vi "Add_Orig_results_filename.vi"() -> ()   [LabVIEW 2010]
uses:
  Controls/File_Selector_Type.ctl
panel:
  in  "Previous Choice":path
  out "Files Processed":i32(slide) scale=0.0..95.0
  out "Current Filename":path
  in  "Search String":string
  in  "At Dialog Prompt Add Metadata to:":T1
  in  "stop":bool
  out "Index":i32=22
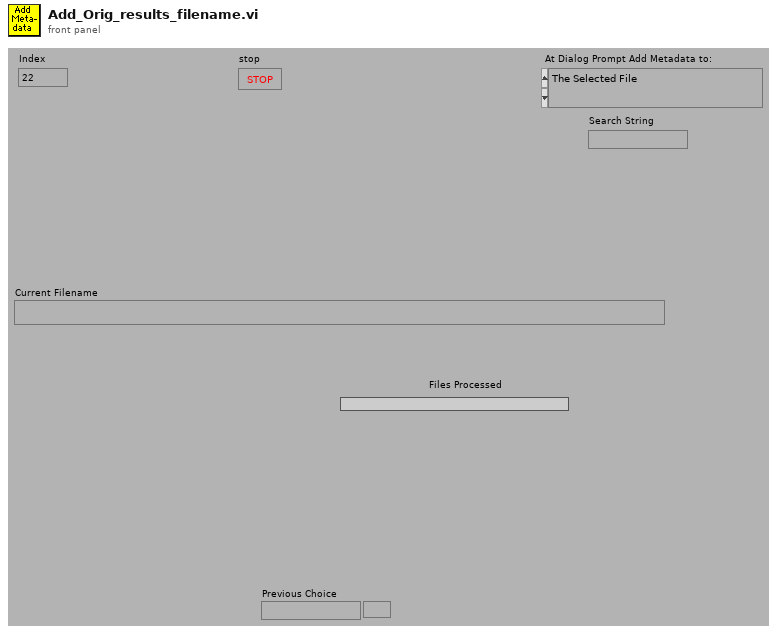
[diagram p1: front panel]
types:
  T1 = typedef "File_Selector_Type.ctl" = enum16{"The Selected File", "The Selected Folder", "Files containing the search string in the selected folder", "All files listed in selected file"}
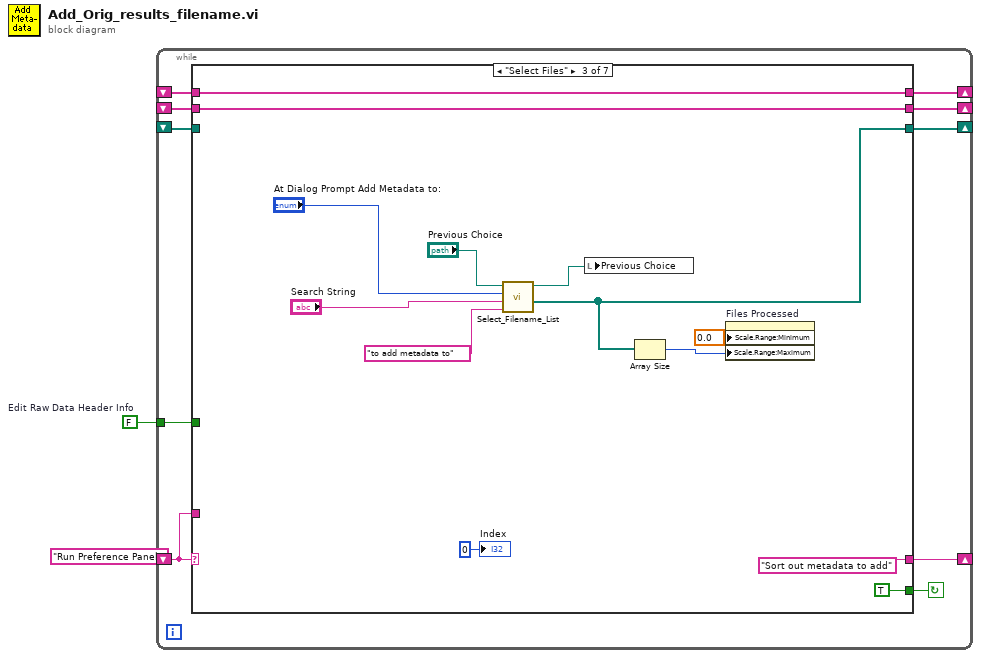
[diagram p0: block diagram]
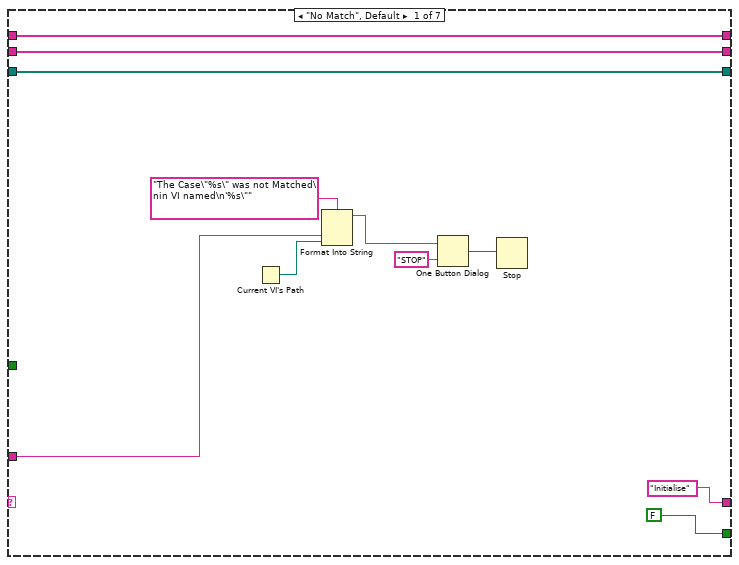
[diagram p2: hidden frame]
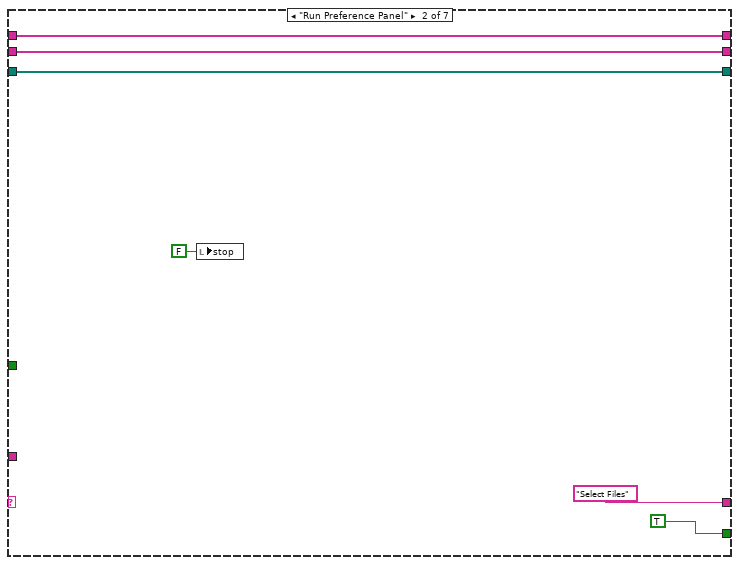
[diagram p3: hidden frame]
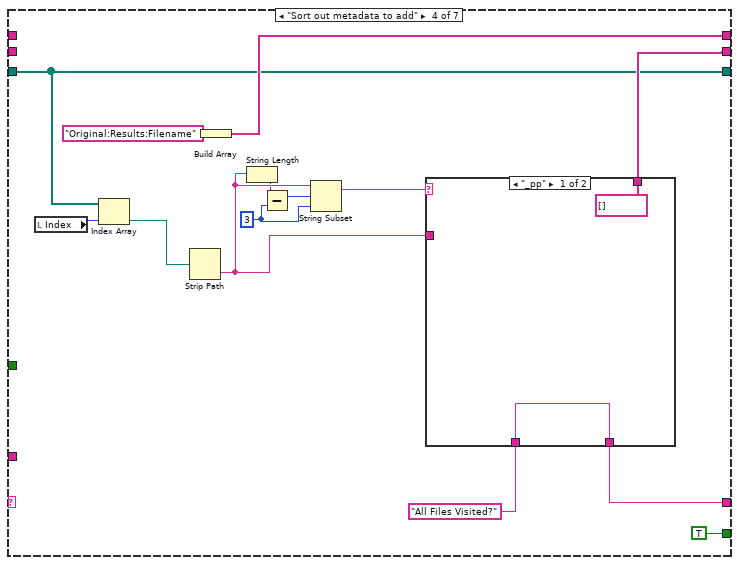
[diagram p4: hidden frame]
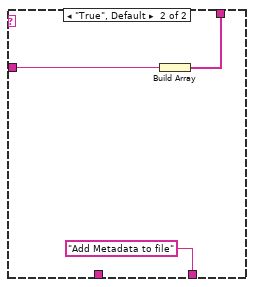
[diagram p5: hidden frame]
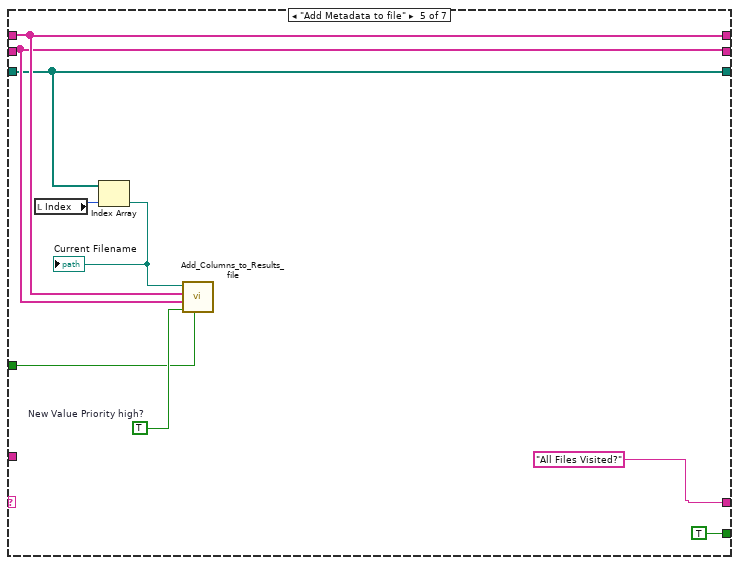
[diagram p6: hidden frame]
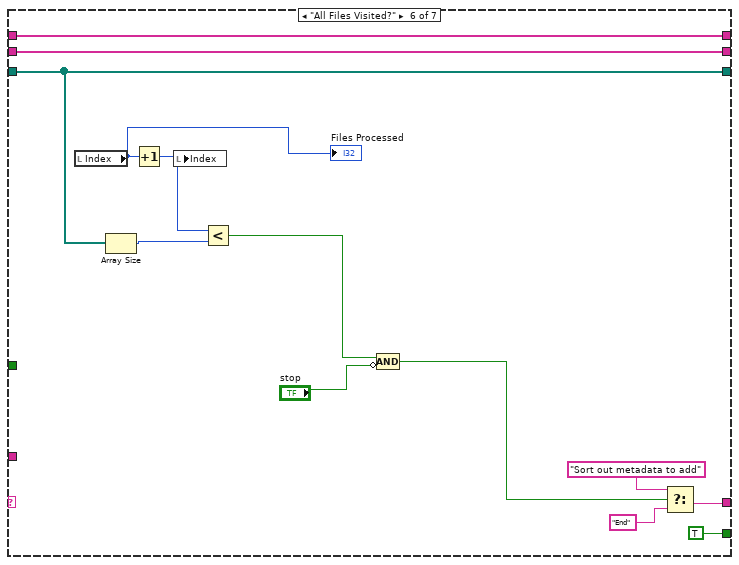
[diagram p7: hidden frame]
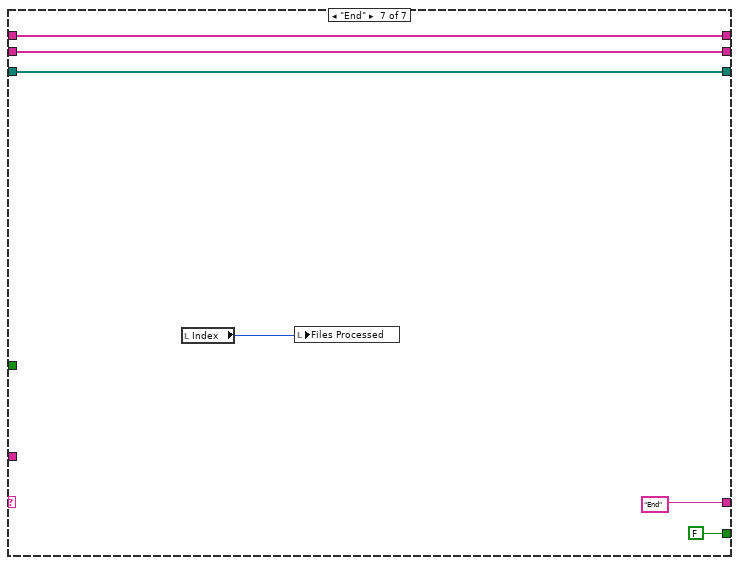
[diagram p8: hidden frame]
diagram:
  w1 = FALSE  # Edit Raw Data Header Info
  n1 = while {
    tunnel: w1 -> [w3]
    shift-left: _ -> [w4]
    shift-right: [w5] -> _
    shift-left: _ -> [w7]
    shift-right: [w6] -> _
    shift-left: _ -> [w9]
    shift-right: [w10] -> _
    shift-left: "Run Preference Panel" -> [w11]
    shift-right: [w12] -> _
    stop <- w8 continue-if-true
    n2 = case shown="\"Select Files\"" w11 {
      tunnel: [FALSE TRUE TRUE TRUE TRUE TRUE FALSE] -> w8
      tunnel: ["Initialise" "Select Files" "Sort out metadata to add" w52 "All Files Visited?" w71 "End"] -> w12
      tunnel: w11 -> [w18 _ _ _ _ _ _]
      tunnel: [w15 w28 w34 w50 w63 w83 w86] -> w10
      tunnel: w9 -> [w15 w28 _ w50 w63 w83 w86]
      tunnel: w7 -> [w14 w26 w37 _ w66 w78 w89]
      tunnel: [w14 w26 w37 w54 w66 w78 w89] -> w6
      tunnel: [w13 w25 w41 w53 w65 w77 w88] -> w5
      tunnel: w4 -> [w13 w25 w41 _ w65 w77 w88]
      tunnel: w3 -> [_ _ _ _ w64 _ _]
      frame "No Match", Default {
        n3 = Current VI's Path() -> (path=w17:path)
        n4 = Format Into String(format string="The Case\"%s\" was not Matched\nin VI named\n'%s\"" ("Format String"), w18, w17) -> (resulting string=w21:string)  [unwired: 2 in, 1 out]
        n5 = One Button Dialog(message=w21, button name ("OK")="STOP") -> (true=w19:bool)
        n6 = Stop(stop? (T)=w19) -> ()
      }
      frame "Run Preference Panel" {
        n7 = local write "stop"(FALSE ("stop")) -> ()
      }
      frame "Select Files" {
        n8 = call "Select_Filename_List.vi"("File Type"="to add metadata to", "Search String"="Search String", "At Dialog Prompt Post Process"="At Dialog Prompt Add Metadata to:", "Previous Choice"="Previous Choice") -> ("Selected files"=w34:path[], "Choosen path"=w31:path)  [unwired: 2 in, 1 out]
        n9 = local write "Previous Choice"(w31) -> ()
        n10 = Array Size(array=w34) -> (size(s)=w33:i32)
        n11 = property on="Files Processed" class="Slide (strict)"("Scale.Range:Minimum"=0.0, "Scale.Range:Maximum"=w33) -> ()  [unwired: 2 in, 2 out]
        "Index" <- 0 ("Index")
      }
      frame "Sort out metadata to add" {
        w45 = 3 ("length (rest)")
        n12 = local read "Index"() -> (w55:i32)
        n13 = Index Array(array=w50, index=w55) -> (element=w49:path)
        n14 = Strip Path(path=w49) -> (name=w47:string)  [unwired: 1 out]
        n15 = Build Array("Original:Results:Filename") -> (w54:string[])
        n16 = String Length(string=w47) -> (length=w46:i32)
        n17 = Subtract(x=w46, y=w45) -> (x-y=w44:i32)
        n18 = String Subset(string=w47, offset (0)=w44, length (rest)=w45) -> (substring=w43:string)
        n19 = case shown="\"_pp\"" w43 {
          tunnel: [string[] [] w59] -> w53
          tunnel: [w57 "Add Metadata to file"] -> w52
          tunnel: "All Files Visited?" -> [w57 _]
          tunnel: w47 -> [_ w60]
          frame "_pp" {
          }
          frame "True", Default {
            n20 = Build Array(w60) -> (w59:string[])
          }
        }
      }
      frame "Add Metadata to file" {
        w67 = TRUE  # New Value Priority high?
        n21 = local read "Index"() -> (w68:i32)
        n22 = Index Array(array=w63, index=w68) -> (element=w69:path)
        "Current Filename" <- w69
        n23 = call "Add_Columns_to_Results_file.vi"("Edit Raw Data Header Info"=w64, "New Value Priority high?"=w67, "New Values In"=w65, "New Chs In"=w66, "Data filename"=w69) -> ()  [unwired: 5 out]
      }
      frame "All Files Visited?" {
        n24 = local read "Index"() -> (w76:i32)
        "Files Processed" <- w76
        n25 = Array Size(array=w83) -> (size(s)=w81:i32)
        n26 = Increment(x=w76) -> (x+1=w82:i32)
        n27 = local write "Index"(w82) -> ()
        n28 = Less?(x=w82, y=w81) -> (x < y?=w79:bool)
        n29 = Compound Arithmetic op=AND(w79, invert "stop") -> (w74:bool)
        n30 = Select(t="Sort out metadata to add", s=w74, f="End") -> (s? t:f=w71:string)
      }
      frame "End" {
        n31 = local read "Index"() -> (w84:i32)
        n32 = local write "Files Processed"(w84) -> ()
      }
    }
  }
